vi "S2C_M2p5942_Proc_Globals.vi"() -> ()   [LabVIEW 2024]
panel:
  out "Running?":bool
  out "Memory":u32
  out "CH Mask":u32
  in  "AI Details":T1
  in  "CardInfo":cluster{"Card Handle":u64, "Error Code":u32}
  in  "5942-Visa":refnum<visa-resource-name>
  out "5942-Refs":string[][](array[string])
  in  "5942-VI":refnum<vi>
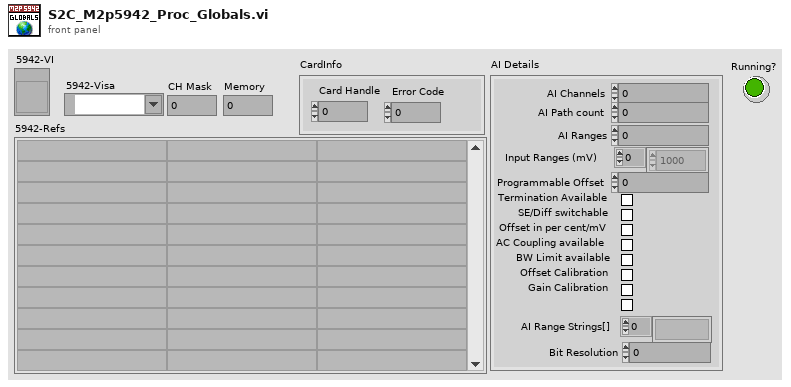
[diagram p1: front panel]
types:
  T1 = cluster{"AI Channels":i32, "AI Ranges":i32, "Input Ranges (mV)":i32[], "Programmable Offset":i32, "Termination Available":bool, "SE/Diff switchable":bool, "Offset in per cent/mV":bool, "Offset Calibration":bool, "Gain Calibration":bool, "Offset with open inputs":bool, "AI Range Strings[]":string[], "Bit Resolution":i32, "AC Coupling available":bool, "BW Limit available":bool, "AI Path count":i32}
diagram:
